vi "Write Build Spec Type.vi"(8 "error in (no error)":errorcluster, 10 "Build Spec GUID":string, 11 "NI Build Specification_LV in":refnum<class "NI Build Specification_LV.lvclass">) -> (0 "error out":errorcluster, 3 "NI Build Specification_LV out":refnum<class "NI Build Specification_LV.lvclass">)   [LabVIEW 2017, in "CL_G3_VIComponentBuilder.lvlib" / "NI Build Specification_LV.lvclass"]
uses:
  NI Build Specification_LV.lvclass
  NI Build Specification_LV.lvclass/NI Build Specification_LV.ctl
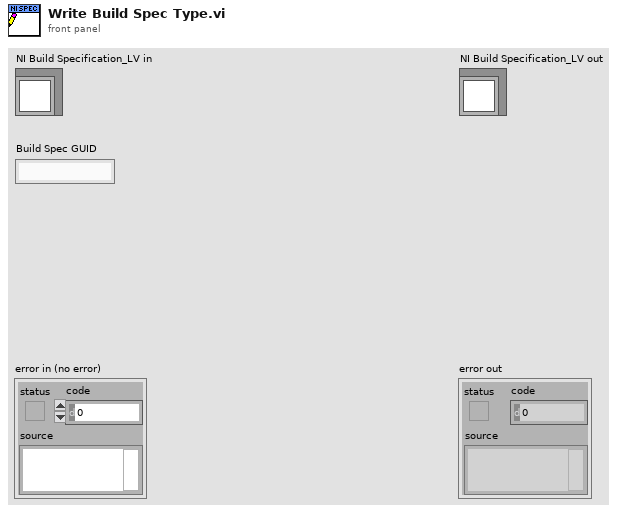
[diagram p1: front panel]
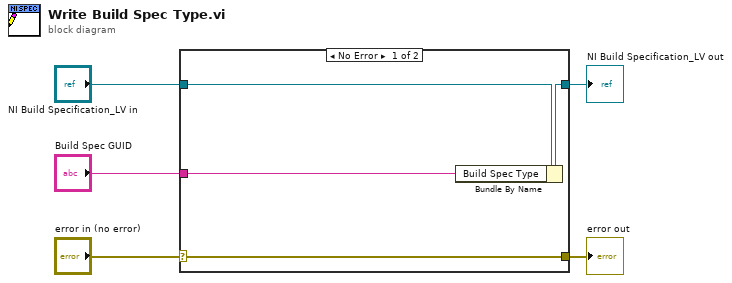
[diagram p0: block diagram]
diagram:
  n1 = case shown="No Error" "error in (no error)" {
    selector: "error in (no error)" -> [w9 w10]
    tunnel: [w9 w10] -> w4
    tunnel: [w7 w11] -> w2
    tunnel: "NI Build Specification_LV in" -> [w8 w11]
    tunnel: "Build Spec GUID" -> [w6 _]
    frame No Error {
      n2 = Bundle By Name(cluster=w8, "Build Spec Type"=w6) -> (w7:refnum<class "NI Build Specification_LV.lvclass">)
    }
    frame Error {
    }
  }
  "error out" <- w4
  "NI Build Specification_LV out" <- w2
